vi "im_gen.vi"() -> ()   [LabVIEW 2009]
panel:
  out "Tamaño de franja":i32
  in  "Coordinates (screen)":cluster{"X Position":i32, "Y Position":i32}={"X Position"=1912, "Y Position"=-30}
  in  "Altura":i32=768 min=0 max=2000
  in  "Ancho":i32=1024
  in  "Nivel de Gris":u8(slide) scale=0.0..255.0
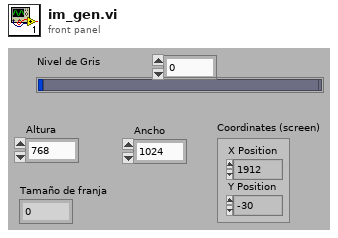
[diagram p1: front panel]
types:
  T1 = typedef "Image Type" = u32
  T2 = typedef "IMAQ Image.ctl" = refnum<image>
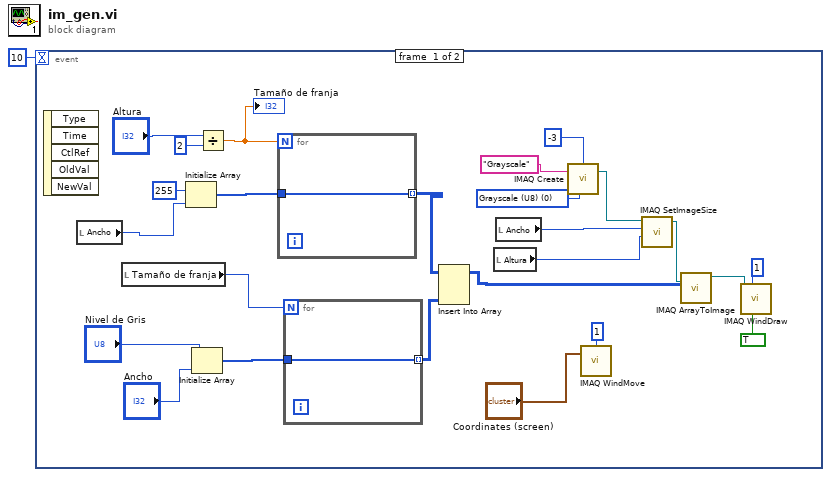
[diagram p0: block diagram]
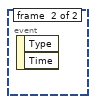
[diagram p2: hidden frame]
diagram:
  n1 = event shown="[1] Timeout" {
    selector: _ -> [_ _]
    dyn-events: _ -> [_ _]
    timeout: 10 -> [_ _]
    event #0 {
      w17 = T1 0 items=["Grayscale (U8)", "Grayscale (I16)", "Grayscale (SGL)", "Complex (CSG)", "RGB (U32)", "HSL (U32)", "RGB (U64)"] ("Image Type")
      n2 = event-data() -> ()  [unwired: 1 in, 5 out]
      n3 = local read "Ancho"() -> (w21:i32)
      n4 = local read "Tamaño de franja"() -> (w2:i32)
      n5 = Initialize Array(u8 255 ("element"), w21) -> (w23:u8[])
      n6 = Initialize Array("Nivel de Gris", "Ancho") -> (w26:u8[])
      n7 = Divide(x="Altura", y=2) -> (x/y=w3:dbl)
      "Tamaño de franja" <- w3
      n8 = for {
        N: w3 -> [_]
        tunnel: w23 -> [w27]
        tunnel: [w27] -> w20 mode=indexing
      }
      n9 = for {
        N: w2 -> [_]
        tunnel: w26 -> [w28]
        tunnel: [w28] -> w19 mode=indexing
      }
      n10 = Insert Into Array(array=w20, new element=w19) -> (w13:u8[][])  [unwired: 2 in]
      n11 = local read "Altura"() -> (w10:i32)
      n12 = local read "Ancho"() -> (w9:i32)
      n13 = call "IMAQ Create"("Border Size"=-3, "Image Name"="Grayscale", "Image Type"=w17) -> ("New Image"=w12:T2)  [unwired: 2 in, 1 out]
      n14 = call "IMAQ WindMove"("Window Number (0...15)"=1, "Coordinates (screen)"="Coordinates (screen)") -> ()  [unwired: 3 in, 2 out]
      n15 = call "IMAQ SetImageSize"("Y Resolution"=w10, "X Resolution"=w9, "Image"=w12) -> ("Image Out"=w11:T2)  [unwired: 2 in, 1 out]
      n16 = call "IMAQ ArrayToImage"("Image Pixels (U8)"=w13, "Image"=w11) -> ("Image Out"=w16:T2)  [unwired: 8 in, 1 out]
      n17 = call "IMAQ WindDraw"("Resize to Image Size? (Y)"=TRUE, "Window Number (0...15)"=1, "Image"=w16) -> ()  [unwired: 7 in, 2 out]
    }
    event #1 {
      n18 = event-data() -> ()  [unwired: 1 in, 2 out]
    }
  }
